vi "WritePanelData_Setup.vi"(8 "error in (no error)":errorcluster, 11 "Maui.Test.DefaultDirectory in":refnum<class "Maui.Test.DefaultDirectory.lvclass">) -> (0 "error out":errorcluster, 3 "Maui.Test.DefaultDirectory out":refnum<class "Maui.Test.DefaultDirectory.lvclass">)   [LabVIEW 2019, in "Maui.Test.DefaultDirectory.lvclass"]
uses:
  Maui.Test.DefaultDirectory.lvclass
  lvsrc/Maui 1.0/SMO.UI.MAUI/SMO.UI.MAUI.lvclass
  lvsrc/Maui 1.0/SMO.UI.MAUI/Typedefs/PanelData.ctl
  C:/Users/Patrick/Documents/GitHub/MAUI-Engine/lvsrc/Maui 1.0/SMO.UI.MAUI/SMO.UI.MAUI.lvclass
  C:/Program Files (x86)/National Instruments/LabVIEW 2019/vi.lib/JKI/JKI SMO/SMO.UI/SMO.UI.lvclass
  C:/Program Files (x86)/National Instruments/LabVIEW 2019/vi.lib/JKI/JKI SMO/SMO/SMO.lvclass
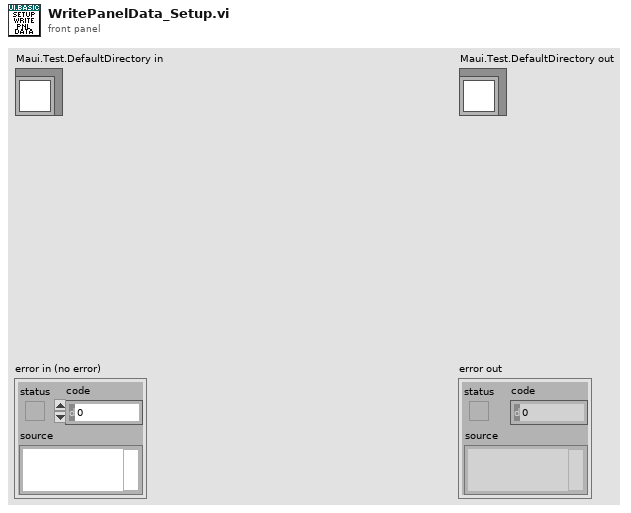
[diagram p1: front panel]
types:
  T1 = typedef "SMO.UI.MAUI.lvclass/PanelData.ctl" = cluster{"SubPanel":refnum<vi>, "Ring":refnum<vi>, "Active":i32}
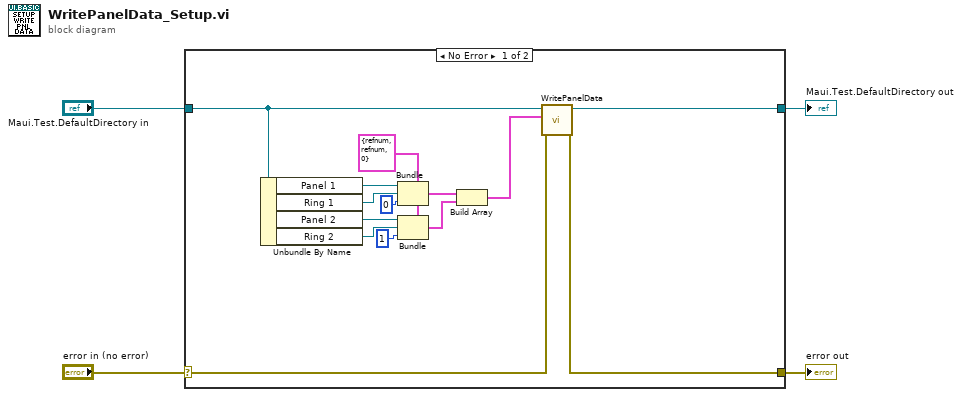
[diagram p0: block diagram]
diagram:
  n1 = case shown="No Error" "error in (no error)" {
    selector: "error in (no error)" -> [w6 w20]
    tunnel: [w5 w20] -> w3
    tunnel: [w8 w19] -> w1
    tunnel: "Maui.Test.DefaultDirectory in" -> [w7 w19]
    frame No Error {
      w16 = T1 {"SubPanel"=refnum, "Ring"=refnum, "Active"=0} ("Panel")
      n2 = Unbundle By Name(w7) -> ("Panel 1"=w9:refnum<vi>, "Ring 1"=w18:refnum<vi>, "Panel 2"=w15:refnum<vi>, "Ring 2"=w10:refnum<vi>)
      n3 = Bundle(cluster=w16, "SubPanel"=w9, "Ring"=w18, "Active"=0) -> (w13:T1)
      n4 = Bundle(cluster=w16, "SubPanel"=w15, "Ring"=w10, "Active"=1) -> (w12:T1)
      n5 = Build Array(w13, w12) -> (w11:T1[])
      n6 = call "WritePanelData.vi"("error in (no error)"=w6, "Panel Data Array"=w11, "MAUI in"=w7) -> ("error out"=w5:errorcluster, "MAUI out"=w8:refnum<class "Maui.Test.DefaultDirectory.lvclass">)  [unwired: 7 in]
    }
    frame Error {
    }
  }
  "error out" <- w3
  "Maui.Test.DefaultDirectory out" <- w1
